vi "Plus.vi"(10 "Y":i32, 11 "X":i32) -> (3 "Result":i32)   [LabVIEW 2015, in "Color Test.lvclass"]
uses:
  Color Test.lvclass
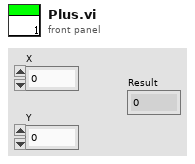
[diagram p1: front panel]
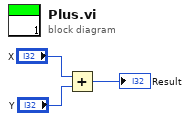
[diagram p0: block diagram]
diagram:
  n1 = Add(x="X", y="Y") -> (x+y=→"Result":i32)
